vi "PID FRC form.vi"(4 "reinitialize? (F)":bool, 5 "output range":cluster{"output high":dbl, "output low":dbl}={"output high"=1.0, "output low"=-1.0} {"output low" format="%.2f"; "output high" format="%.2f"}, 6 "dt (s)":dbl=-1.0 format="%.3f", 7 "setpoint":dbl format="%.2f", 8 "d smoothing":dbl=nan format="%.2f", 9 "Arbitrary Bias":dbl=1.5000000000000002, 10 "process variable":dbl format="%.2f", 11 "PIDF gains":T1={"proportional (Kp)"=1.0, "integral (Ki)"=0.0, "derivative (Kd)"=0.0, "feedFwd (Kff)"=0.0} {"feedFwd (Kff)" format="%.3f"; "derivative (Kd)" format="%.3f"; "integral (Ki)" format="%.3f"; "proportional (Kp)" format="%.3f"}) -> (0 "dt out (s)":dbl format="%.3f", 1 "Err/Out Chart":cluster{dbl, dbl}(graph), 2 "SP/PV Chart":cluster{"setpoint":dbl, "process variable":dbl}(graph), 3 "output":dbl format="%.2f")   [LabVIEW 2020]
doc: "Implements a PID that meets FRC needs. It is in parallel form (Kp, Ki, Kd) and includes an arbitrary feedforward that is added to the output.\nThe PID algorithm features control output range limiting with integrator anti-windup and bumpless controller output for PID gain changes. The d smoothing (0-1) can help avoid oscillations due to stronger d terms."
uses:
  <vilib>/addons/control/pid/pid.llb/PID Structure.ctl
  <vilib>/addons/control/pid/pid.llb/PID Structure Conversion (DBL).vi
  <vilib>/addons/control/pid/pid.llb/PID Advanced (DBL).vi
  <vilib>/addons/control/pid/NI_PID_pid.lvlib
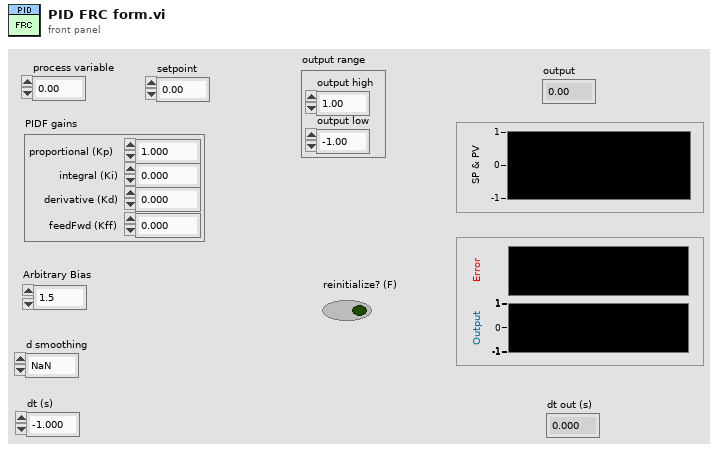
[diagram p1: front panel]
types:
  T1 = cluster{"proportional (Kp)":dbl, "integral (Ki)":dbl, "derivative (Kd)":dbl, "feedFwd (Kff)":dbl}
  T2 = typedef "NI_PID_pid.lvlib/PID Structure.ctl" = u16
  T3 = cluster{"proportional gain (Kc)":dbl, "integral time (Ti, min)":dbl, "derivative time (Td, min)":dbl}
  T4 = cluster{"proportional gain (Kc)":bool, "integral time (Ti, min)":bool, "derivative time (Td, min)":bool}
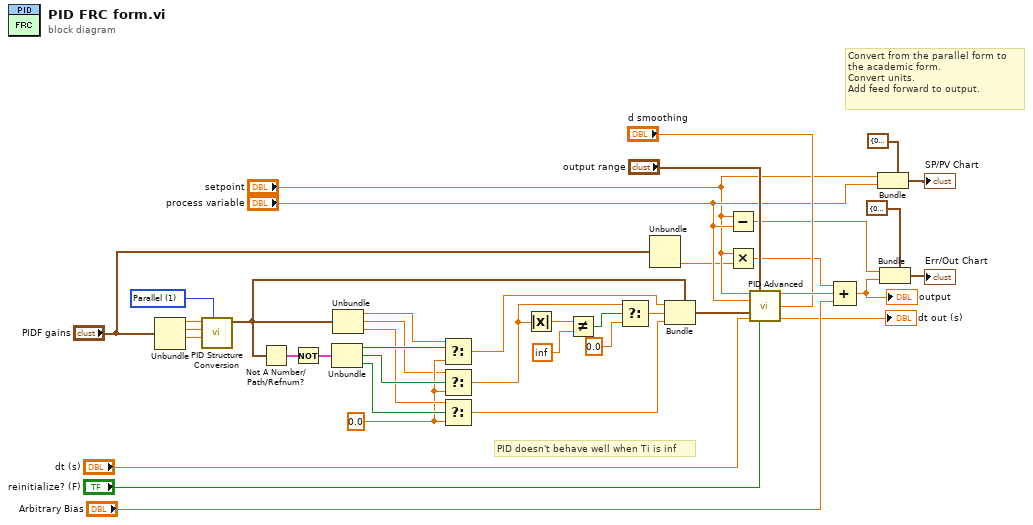
[diagram p0: block diagram]
diagram:
  w25 = 0.0
  w41 = T2 1 items=["Academic (Standard)", "Parallel", "Series"] ("PID structure")
  # "PID doesn't behave well when Ti is inf"
  # "Convert from the parallel form to\nthe academic form.\nConvert units.\nAdd feed forward to output."
  n1 = Unbundle("PIDF gains") -> ("proportional (Kp)"=w40:dbl, "integral (Ki)"=w39:dbl, "derivative (Kd)"=w38:dbl)  [unwired: 1 out]
  n2 = call-poly <vilib>:"PID Structure Conversion.vi"("PID structure"=w41, "derivative"=w38, "integral"=w39, "proportional"=w40) -> ("PID gains"=w33:T3)  [unwired: 7 in]
  n3 = Not A Number/Path/Refnum?(number/path/refnum=w33) -> (NaN/Path/Refnum?=w32:T4)
  n4 = Not(x=w32) -> (.not. x?=w30:T4)
  n5 = Unbundle(w30) -> ("proportional gain (Kc)"=w31:bool, "integral time (Ti, min)"=w28:bool, "derivative time (Td, min)"=w27:bool)
  n6 = Unbundle(w33) -> ("proportional gain (Kc)"=w29:dbl, "integral time (Ti, min)"=w24:dbl, "derivative time (Td, min)"=w26:dbl)
  n7 = Select(t=w29, s=w31, f=w25) -> (s? t:f=w23:dbl)
  n8 = Select(t=w24, s=w28, f=w25) -> (s? t:f=w21:dbl)
  n9 = Select(t=w26, s=w27, f=w25) -> (s? t:f=w22:dbl)
  n10 = Absolute Value(x=w21) -> (abs(x)=w36:dbl)
  n11 = Not Equal?(x=w36, y=inf) -> (x != y?=w35:bool)
  n12 = Select(t=w21, s=w35, f=0.0) -> (s? t:f=w13:dbl)
  n13 = Unbundle("PIDF gains") -> ("feedFwd (Kff)"=w2:dbl)  [unwired: 3 out]
  n14 = Bundle(cluster=w33, "proportional gain (Kc)"=w23, "integral time (Ti, min)"=w13, "derivative time (Td, min)"=w22) -> (w17:T3)
  n15 = Subtract(x="setpoint", y="process variable") -> (x-y=w7:dbl)
  n16 = Multiply(x="setpoint", y=w2) -> (x*y=w1:dbl)
  n17 = call-poly <vilib>:"PID Advanced.vi"("setpoint"="setpoint", "output range"="output range", "process variable"="process variable", "alpha"="d smoothing", "PID gains"=w17, "dt (s)"="dt (s)", "reinitialize? (F)"="reinitialize? (F)") -> ("output"=w15:dbl, "dt out (s)"=→"dt out (s)":dbl)  [unwired: 7 in]
  n18 = Compound Arithmetic op=ADD(w1, w15, "Arbitrary Bias") -> (w8:dbl)
  "output" <- w8
  n19 = Bundle(cluster=cluster{"setpoint":dbl, "process variable":dbl} {"setpoint"=0.0, "process variable"=0.0}, "setpoint"="setpoint", "process variable"="process variable") -> (→"SP/PV Chart":cluster{"setpoint":dbl, "process variable":dbl})
  n20 = Bundle(cluster=cluster{"Error":dbl, "Output":dbl} {"Error"=0.0, "Output"=0.0}, "Error"=w7, "Output"=w8) -> (→"Err/Out Chart":cluster{"Error":dbl, "Output":dbl})
